vi "PicoScope6000aExampleStreamingQueue.vi"() -> ()   [LabVIEW 2015]
doc: "ps6000a Streaming example filling a single set of channel buffers at a time with LabVIEW queues."
uses:
  shared/PicoBuffers.ctl
  <vilib>/Waveform/DWDTOps.llb/DWDT Analog to Digital.vi
  PicoScope6000aLib/PicoScope6000aDigitalChannelSettings.ctl
  PicoScope6000aLib/PicoScope6000aAnalogChannelSettings.ctl
panel:
  in  "Poll Delay %":dbl=1.0 format="%#_13g"
  in  "Poll Holdoff %":dbl=90.0 format="%#_13g"
  out "Port 0":digitalwaveform(graph)={"t0"=timestamp(0 s since 1904-01-01), "dt"=1.004800013071339e-06, "Y"={"transitions"=[], "data"=[]}}
  out "Analog Channels":cluster{i32, dbl, "Data":dbl[]}[](graph)
  in  "Write ChA to file":bool
  out "Queue depth":i32(graph)
  out "queue depth":i32
  in  "Data file":path=path "PicoScope6000aExampleStreaming ChA Data"
  out "Max ADC value":i16
  out "DownSample Interval (sec)":dbl=1.0000000130088963e-06 format="%#.5p"
  out "Chunk time":u32
  out "Elapsed time":dbl
  in  "Auto Stop":bool
  in  "Apply Settings":bool
  in  "Channels":T1={"Channel A Settings "={"Enabled"=TRUE, "Coupling"=1, "Range"=0, "Analogue Offset"=0.0, "BandWidth"=0}, "Channel B Settings "={"Enabled"=FALSE, "Coupling"=1, "Range"=0, "Analogue Offset"=0.0, "BandWidth"=0}, "Channel C Settings "={"Enabled"=FALSE, "Coupling"=1, "Range"=0, "Analogue Offset"=0.0, "BandWidth"=0}, "Channel D Settings "={"Enabled"=FALSE, "Coupling"=1, "Range"=0, "Analogue Offset"=0.0, "BandWidth"=0}, "Channel E Settings "={"Enabled"=FALSE, "Coupling"=1, "Range"=0, "Analogue Offset"=0.0, "BandWidth"=0}, "Channel F Settings "={"Enabled"=FALSE, "Coupling"=1, "Range"=0, "Analogue Offset"=0.0, "BandWidth"=0}, "Channel G Settings "={"Enabled"=FALSE, "Coupling"=1, "Range"=0, "Analogue Offset"=0.0, "BandWidth"=0}, "Channel H Settings "={"Enabled"=FALSE, "Coupling"=1, "Range"=0, "Analogue Offset"=0.0, "BandWidth"=0}} {"Channel H Settings"."BandWidth" items=["Full"=0, "100kHz"=100000, "20kHz"=200000, "1MHz"=1000000, "20MHz"=20000000, "25MHz"=25000000, "50MHz"=50000000, "200MHz"=200000000, "250MHz"=250000000, "500MHz"=500000000]; "Channel H Settings"."Range" items=["10mV"=0, "20mV"=1, "50mV"=2, "100mV"=3, "200mV"=4, "500mV"=5, "1V"=6, "2V"=7, "5V"=8, "10V"=9, "20V"=10, "50V"=11, "100V"=12, "200V"=13, "x10_Probe_100mV"=32, "x10_Probe_200mV"=33, "x10_Probe_500mV"=34, "x10_Probe_1V"=35, "x10_Probe_2V"=36, "x10_Probe_5V"=37, "x10_Probe_10V"=38, "x10_Probe_20V"=39, "x10_Probe_50V"=40, "x10_Probe_100V"=41, "x10_Probe_200V"=42, "x10_Probe_500V"=43, "CURRENT_CLAMP_60A_2A"=10500, "CURRENT_CLAMP_60A_5A"=10501, "CURRENT_CLAMP_60A_10A"=10502, "CURRENT_CLAMP_60A_20A"=10503, "CURRENT_CLAMP_60A_50A"=10504, "CURRENT_CLAMP_60A_60A"=10505, "CURRENT_CLAMP_60A_V2_0_5A"=10600, "CURRENT_CLAMP_60A_V2_1A"=10601, "CURRENT_CLAMP_60A_V2_2A"=10602, "CURRENT_CLAMP_60A_V2_5A"=10603, "CURRENT_CLAMP_60A_V2_10A"=10604, "CURRENT_CLAMP_60A_V2_20A"=10605, "CURRENT_CLAMP_60A_V2_50A"=10606, "CURRENT_CLAMP_60A_V2_60A"=10607, "RESISTANCE_LEAD_NEG5_TO_20OHM"=7000, "RESISTANCE_LEAD_NEG50_TO_200OHM"=7001, "RESISTANCE_LEAD_NEG500_TO_2KOHM"=7002, "RESISTANCE_LEAD_NEG5K_TO_20KOHM"=7003, "RESISTANCE_LEAD_NEG50K_TO_LEAD_200KOHM"=7004, "RESISTANCE_LEAD_NEG500K_TO_LEAD_2MOHM"=7005, "RESISTANCE_LEAD_DIODE_TEST"=7006, "HT_NEG3_TO_5KV"=8950, "HT_NEG3_TO_10KV"=8951, "HT_NEG5_TO_20KV"=8952, "HT_NEG5_TO_50KV"=8953, "HT_NEG5_TO_100KV"=8954, "HT_NEG3_TO_5KV_INVERTED"=8955, "HT_NEG3_TO_10KV_INVERTED"=8956, "HT_NEG5_TO_20KV_INVERTED"=8957, "HT_NEG5_TO_50KV_INVERTED"=8958, "HT_NEG5_TO_100KV_INVERTED"=8959, "TEMPERATURE_NEG50_TO_150DEGC"=9000, "PRESSURE_SENSOR_-100k-150k_PASCALS"=9100, "PRESSURE_SENSOR_-100k_TO_400k_PASCALS"=9101, "PRESSURE_SENSOR_-200k_TO_800k_PASCALS"=9102, "PRESSURE_SENSOR_-400k_TO_1600k_PASCALS"=9103, "PRESSURE_SENSOR_-400k_TO_3400k_PASCALS"=9104, "PRESSURE_SENSOR_-150k_TO_1350k_PASCALS"=9105]; "Channel H Settings"."Coupling" items=["AC"=0, "DC 1M Ohm"=1, "DC 50 Ohm"=50]; "Channel G Settings"."BandWidth" items=["Full"=0, "100kHz"=100000, "20kHz"=200000, "1MHz"=1000000, "20MHz"=20000000, "25MHz"=25000000, "50MHz"=50000000, "200MHz"=200000000, "250MHz"=250000000, "500MHz"=500000000]; "Channel G Settings"."Range" items=["10mV"=0, "20mV"=1, "50mV"=2, "100mV"=3, "200mV"=4, "500mV"=5, "1V"=6, "2V"=7, "5V"=8, "10V"=9, "20V"=10, "50V"=11, "100V"=12, "200V"=13, "x10_Probe_100mV"=32, "x10_Probe_200mV"=33, "x10_Probe_500mV"=34, "x10_Probe_1V"=35, "x10_Probe_2V"=36, "x10_Probe_5V"=37, "x10_Probe_10V"=38, "x10_Probe_20V"=39, "x10_Probe_50V"=40, "x10_Probe_100V"=41, "x10_Probe_200V"=42, "x10_Probe_500V"=43, "CURRENT_CLAMP_60A_2A"=10500, "CURRENT_CLAMP_60A_5A"=10501, "CURRENT_CLAMP_60A_10A"=10502, "CURRENT_CLAMP_60A_20A"=10503, "CURRENT_CLAMP_60A_50A"=10504, "CURRENT_CLAMP_60A_60A"=10505, "CURRENT_CLAMP_60A_V2_0_5A"=10600, "CURRENT_CLAMP_60A_V2_1A"=10601, "CURRENT_CLAMP_60A_V2_2A"=10602, "CURRENT_CLAMP_60A_V2_5A"=10603, "CURRENT_CLAMP_60A_V2_10A"=10604, "CURRENT_CLAMP_60A_V2_20A"=10605, "CURRENT_CLAMP_60A_V2_50A"=10606, "CURRENT_CLAMP_60A_V2_60A"=10607, "RESISTANCE_LEAD_NEG5_TO_20OHM"=7000, "RESISTANCE_LEAD_NEG50_TO_200OHM"=7001, "RESISTANCE_LEAD_NEG500_TO_2KOHM"=7002, "RESISTANCE_LEAD_NEG5K_TO_20KOHM"=7003, "RESISTANCE_LEAD_NEG50K_TO_LEAD_200KOHM"=7004, "RESISTANCE_LEAD_NEG500K_TO_LEAD_2MOHM"=7005, "RESISTANCE_LEAD_DIODE_TEST"=7006, "HT_NEG3_TO_5KV"=8950, "HT_NEG3_TO_10KV"=8951, "HT_NEG5_TO_20KV"=8952, "HT_NEG5_TO_50KV"=8953, "HT_NEG5_TO_100KV"=8954, "HT_NEG3_TO_5KV_INVERTED"=8955, "HT_NEG3_TO_10KV_INVERTED"=8956, "HT_NEG5_TO_20KV_INVERTED"=8957, "HT_NEG5_TO_50KV_INVERTED"=8958, "HT_NEG5_TO_100KV_INVERTED"=8959, "TEMPERATURE_NEG50_TO_150DEGC"=9000, "PRESSURE_SENSOR_-100k-150k_PASCALS"=9100, "PRESSURE_SENSOR_-100k_TO_400k_PASCALS"=9101, "PRESSURE_SENSOR_-200k_TO_800k_PASCALS"=9102, "PRESSURE_SENSOR_-400k_TO_1600k_PASCALS"=9103, "PRESSURE_SENSOR_-400k_TO_3400k_PASCALS"=9104, "PRESSURE_SENSOR_-150k_TO_1350k_PASCALS"=9105]; "Channel G Settings"."Coupling" items=["AC"=0, "DC 1M Ohm"=1, "DC 50 Ohm"=50]; "Channel F Settings"."BandWidth" items=["Full"=0, "100kHz"=100000, "20kHz"=200000, "1MHz"=1000000, "20MHz"=20000000, "25MHz"=25000000, "50MHz"=50000000, "200MHz"=200000000, "250MHz"=250000000, "500MHz"=500000000]; "Channel F Settings"."Range" items=["10mV"=0, "20mV"=1, "50mV"=2, "100mV"=3, "200mV"=4, "500mV"=5, "1V"=6, "2V"=7, "5V"=8, "10V"=9, "20V"=10, "50V"=11, "100V"=12, "200V"=13, "x10_Probe_100mV"=32, "x10_Probe_200mV"=33, "x10_Probe_500mV"=34, "x10_Probe_1V"=35, "x10_Probe_2V"=36, "x10_Probe_5V"=37, "x10_Probe_10V"=38, "x10_Probe_20V"=39, "x10_Probe_50V"=40, "x10_Probe_100V"=41, "x10_Probe_200V"=42, "x10_Probe_500V"=43, "CURRENT_CLAMP_60A_2A"=10500, "CURRENT_CLAMP_60A_5A"=10501, "CURRENT_CLAMP_60A_10A"=10502, "CURRENT_CLAMP_60A_20A"=10503, "CURRENT_CLAMP_60A_50A"=10504, "CURRENT_CLAMP_60A_60A"=10505, "CURRENT_CLAMP_60A_V2_0_5A"=10600, "CURRENT_CLAMP_60A_V2_1A"=10601, "CURRENT_CLAMP_60A_V2_2A"=10602, "CURRENT_CLAMP_60A_V2_5A"=10603, "CURRENT_CLAMP_60A_V2_10A"=10604, "CURRENT_CLAMP_60A_V2_20A"=10605, "CURRENT_CLAMP_60A_V2_50A"=10606, "CURRENT_CLAMP_60A_V2_60A"=10607, "RESISTANCE_LEAD_NEG5_TO_20OHM"=7000, "RESISTANCE_LEAD_NEG50_TO_200OHM"=7001, "RESISTANCE_LEAD_NEG500_TO_2KOHM"=7002, "RESISTANCE_LEAD_NEG5K_TO_20KOHM"=7003, "RESISTANCE_LEAD_NEG50K_TO_LEAD_200KOHM"=7004, "RESISTANCE_LEAD_NEG500K_TO_LEAD_2MOHM"=7005, "RESISTANCE_LEAD_DIODE_TEST"=7006, "HT_NEG3_TO_5KV"=8950, "HT_NEG3_TO_10KV"=8951, "HT_NEG5_TO_20KV"=8952, "HT_NEG5_TO_50KV"=8953, "HT_NEG5_TO_100KV"=8954, "HT_NEG3_TO_5KV_INVERTED"=8955, "HT_NEG3_TO_10KV_INVERTED"=8956, "HT_NEG5_TO_20KV_INVERTED"=8957, "HT_NEG5_TO_50KV_INVERTED"=8958, "HT_NEG5_TO_100KV_INVERTED"=8959, "TEMPERATURE_NEG50_TO_150DEGC"=9000, "PRESSURE_SENSOR_-100k-150k_PASCALS"=9100, "PRESSURE_SENSOR_-100k_TO_400k_PASCALS"=9101, "PRESSURE_SENSOR_-200k_TO_800k_PASCALS"=9102, "PRESSURE_SENSOR_-400k_TO_1600k_PASCALS"=9103, "PRESSURE_SENSOR_-400k_TO_3400k_PASCALS"=9104, "PRESSURE_SENSOR_-150k_TO_1350k_PASCALS"=9105]; "Channel F Settings"."Coupling" items=["AC"=0, "DC 1M Ohm"=1, "DC 50 Ohm"=50]; "Channel E Settings"."BandWidth" items=["Full"=0, "100kHz"=100000, "20kHz"=200000, "1MHz"=1000000, "20MHz"=20000000, "25MHz"=25000000, "50MHz"=50000000, "200MHz"=200000000, "250MHz"=250000000, "500MHz"=500000000]; "Channel E Settings"."Range" items=["10mV"=0, "20mV"=1, "50mV"=2, "100mV"=3, "200mV"=4, "500mV"=5, "1V"=6, "2V"=7, "5V"=8, "10V"=9, "20V"=10, "50V"=11, "100V"=12, "200V"=13, "x10_Probe_100mV"=32, "x10_Probe_200mV"=33, "x10_Probe_500mV"=34, "x10_Probe_1V"=35, "x10_Probe_2V"=36, "x10_Probe_5V"=37, "x10_Probe_10V"=38, "x10_Probe_20V"=39, "x10_Probe_50V"=40, "x10_Probe_100V"=41, "x10_Probe_200V"=42, "x10_Probe_500V"=43, "CURRENT_CLAMP_60A_2A"=10500, "CURRENT_CLAMP_60A_5A"=10501, "CURRENT_CLAMP_60A_10A"=10502, "CURRENT_CLAMP_60A_20A"=10503, "CURRENT_CLAMP_60A_50A"=10504, "CURRENT_CLAMP_60A_60A"=10505, "CURRENT_CLAMP_60A_V2_0_5A"=10600, "CURRENT_CLAMP_60A_V2_1A"=10601, "CURRENT_CLAMP_60A_V2_2A"=10602, "CURRENT_CLAMP_60A_V2_5A"=10603, "CURRENT_CLAMP_60A_V2_10A"=10604, "CURRENT_CLAMP_60A_V2_20A"=10605, "CURRENT_CLAMP_60A_V2_50A"=10606, "CURRENT_CLAMP_60A_V2_60A"=10607, "RESISTANCE_LEAD_NEG5_TO_20OHM"=7000, "RESISTANCE_LEAD_NEG50_TO_200OHM"=7001, "RESISTANCE_LEAD_NEG500_TO_2KOHM"=7002, "RESISTANCE_LEAD_NEG5K_TO_20KOHM"=7003, "RESISTANCE_LEAD_NEG50K_TO_LEAD_200KOHM"=7004, "RESISTANCE_LEAD_NEG500K_TO_LEAD_2MOHM"=7005, "RESISTANCE_LEAD_DIODE_TEST"=7006, "HT_NEG3_TO_5KV"=8950, "HT_NEG3_TO_10KV"=8951, "HT_NEG5_TO_20KV"=8952, "HT_NEG5_TO_50KV"=8953, "HT_NEG5_TO_100KV"=8954, "HT_NEG3_TO_5KV_INVERTED"=8955, "HT_NEG3_TO_10KV_INVERTED"=8956, "HT_NEG5_TO_20KV_INVERTED"=8957, "HT_NEG5_TO_50KV_INVERTED"=8958, "HT_NEG5_TO_100KV_INVERTED"=8959, "TEMPERATURE_NEG50_TO_150DEGC"=9000, "PRESSURE_SENSOR_-100k-150k_PASCALS"=9100, "PRESSURE_SENSOR_-100k_TO_400k_PASCALS"=9101, "PRESSURE_SENSOR_-200k_TO_800k_PASCALS"=9102, "PRESSURE_SENSOR_-400k_TO_1600k_PASCALS"=9103, "PRESSURE_SENSOR_-400k_TO_3400k_PASCALS"=9104, "PRESSURE_SENSOR_-150k_TO_1350k_PASCALS"=9105]; "Channel E Settings"."Coupling" items=["AC"=0, "DC 1M Ohm"=1, "DC 50 Ohm"=50]; "Channel D Settings"."BandWidth" items=["Full"=0, "100kHz"=100000, "20kHz"=200000, "1MHz"=1000000, "20MHz"=20000000, "25MHz"=25000000, "50MHz"=50000000, "200MHz"=200000000, "250MHz"=250000000, "500MHz"=500000000]; "Channel D Settings"."Range" items=["10mV"=0, "20mV"=1, "50mV"=2, "100mV"=3, "200mV"=4, "500mV"=5, "1V"=6, "2V"=7, "5V"=8, "10V"=9, "20V"=10, "50V"=11, "100V"=12, "200V"=13, "x10_Probe_100mV"=32, "x10_Probe_200mV"=33, "x10_Probe_500mV"=34, "x10_Probe_1V"=35, "x10_Probe_2V"=36, "x10_Probe_5V"=37, "x10_Probe_10V"=38, "x10_Probe_20V"=39, "x10_Probe_50V"=40, "x10_Probe_100V"=41, "x10_Probe_200V"=42, "x10_Probe_500V"=43, "CURRENT_CLAMP_60A_2A"=10500, "CURRENT_CLAMP_60A_5A"=10501, "CURRENT_CLAMP_60A_10A"=10502, "CURRENT_CLAMP_60A_20A"=10503, "CURRENT_CLAMP_60A_50A"=10504, "CURRENT_CLAMP_60A_60A"=10505, "CURRENT_CLAMP_60A_V2_0_5A"=10600, "CURRENT_CLAMP_60A_V2_1A"=10601, "CURRENT_CLAMP_60A_V2_2A"=10602, "CURRENT_CLAMP_60A_V2_5A"=10603, "CURRENT_CLAMP_60A_V2_10A"=10604, "CURRENT_CLAMP_60A_V2_20A"=10605, "CURRENT_CLAMP_60A_V2_50A"=10606, "CURRENT_CLAMP_60A_V2_60A"=10607, "RESISTANCE_LEAD_NEG5_TO_20OHM"=7000, "RESISTANCE_LEAD_NEG50_TO_200OHM"=7001, "RESISTANCE_LEAD_NEG500_TO_2KOHM"=7002, "RESISTANCE_LEAD_NEG5K_TO_20KOHM"=7003, "RESISTANCE_LEAD_NEG50K_TO_LEAD_200KOHM"=7004, "RESISTANCE_LEAD_NEG500K_TO_LEAD_2MOHM"=7005, "RESISTANCE_LEAD_DIODE_TEST"=7006, "HT_NEG3_TO_5KV"=8950, "HT_NEG3_TO_10KV"=8951, "HT_NEG5_TO_20KV"=8952, "HT_NEG5_TO_50KV"=8953, "HT_NEG5_TO_100KV"=8954, "HT_NEG3_TO_5KV_INVERTED"=8955, "HT_NEG3_TO_10KV_INVERTED"=8956, "HT_NEG5_TO_20KV_INVERTED"=8957, "HT_NEG5_TO_50KV_INVERTED"=8958, "HT_NEG5_TO_100KV_INVERTED"=8959, "TEMPERATURE_NEG50_TO_150DEGC"=9000, "PRESSURE_SENSOR_-100k-150k_PASCALS"=9100, "PRESSURE_SENSOR_-100k_TO_400k_PASCALS"=9101, "PRESSURE_SENSOR_-200k_TO_800k_PASCALS"=9102, "PRESSURE_SENSOR_-400k_TO_1600k_PASCALS"=9103, "PRESSURE_SENSOR_-400k_TO_3400k_PASCALS"=9104, "PRESSURE_SENSOR_-150k_TO_1350k_PASCALS"=9105]; "Channel D Settings"."Coupling" items=["AC"=0, "DC 1M Ohm"=1, "DC 50 Ohm"=50]; "Channel C Settings"."BandWidth" items=["Full"=0, "100kHz"=100000, "20kHz"=200000, "1MHz"=1000000, "20MHz"=20000000, "25MHz"=25000000, "50MHz"=50000000, "200MHz"=200000000, "250MHz"=250000000, "500MHz"=500000000]; "Channel C Settings"."Range" items=["10mV"=0, "20mV"=1, "50mV"=2, "100mV"=3, "200mV"=4, "500mV"=5, "1V"=6, "2V"=7, "5V"=8, "10V"=9, "20V"=10, "50V"=11, "100V"=12, "200V"=13, "x10_Probe_100mV"=32, "x10_Probe_200mV"=33, "x10_Probe_500mV"=34, "x10_Probe_1V"=35, "x10_Probe_2V"=36, "x10_Probe_5V"=37, "x10_Probe_10V"=38, "x10_Probe_20V"=39, "x10_Probe_50V"=40, "x10_Probe_100V"=41, "x10_Probe_200V"=42, "x10_Probe_500V"=43, "CURRENT_CLAMP_60A_2A"=10500, "CURRENT_CLAMP_60A_5A"=10501, "CURRENT_CLAMP_60A_10A"=10502, "CURRENT_CLAMP_60A_20A"=10503, "CURRENT_CLAMP_60A_50A"=10504, "CURRENT_CLAMP_60A_60A"=10505, "CURRENT_CLAMP_60A_V2_0_5A"=10600, "CURRENT_CLAMP_60A_V2_1A"=10601, "CURRENT_CLAMP_60A_V2_2A"=10602, "CURRENT_CLAMP_60A_V2_5A"=10603, "CURRENT_CLAMP_60A_V2_10A"=10604, "CURRENT_CLAMP_60A_V2_20A"=10605, "CURRENT_CLAMP_60A_V2_50A"=10606, "CURRENT_CLAMP_60A_V2_60A"=10607, "RESISTANCE_LEAD_NEG5_TO_20OHM"=7000, "RESISTANCE_LEAD_NEG50_TO_200OHM"=7001, "RESISTANCE_LEAD_NEG500_TO_2KOHM"=7002, "RESISTANCE_LEAD_NEG5K_TO_20KOHM"=7003, "RESISTANCE_LEAD_NEG50K_TO_LEAD_200KOHM"=7004, "RESISTANCE_LEAD_NEG500K_TO_LEAD_2MOHM"=7005, "RESISTANCE_LEAD_DIODE_TEST"=7006, "HT_NEG3_TO_5KV"=8950, "HT_NEG3_TO_10KV"=8951, "HT_NEG5_TO_20KV"=8952, "HT_NEG5_TO_50KV"=8953, "HT_NEG5_TO_100KV"=8954, "HT_NEG3_TO_5KV_INVERTED"=8955, "HT_NEG3_TO_10KV_INVERTED"=8956, "HT_NEG5_TO_20KV_INVERTED"=8957, "HT_NEG5_TO_50KV_INVERTED"=8958, "HT_NEG5_TO_100KV_INVERTED"=8959, "TEMPERATURE_NEG50_TO_150DEGC"=9000, "PRESSURE_SENSOR_-100k-150k_PASCALS"=9100, "PRESSURE_SENSOR_-100k_TO_400k_PASCALS"=9101, "PRESSURE_SENSOR_-200k_TO_800k_PASCALS"=9102, "PRESSURE_SENSOR_-400k_TO_1600k_PASCALS"=9103, "PRESSURE_SENSOR_-400k_TO_3400k_PASCALS"=9104, "PRESSURE_SENSOR_-150k_TO_1350k_PASCALS"=9105]; "Channel C Settings"."Coupling" items=["AC"=0, "DC 1M Ohm"=1, "DC 50 Ohm"=50]; "Channel B Settings"."BandWidth" items=["Full"=0, "100kHz"=100000, "20kHz"=200000, "1MHz"=1000000, "20MHz"=20000000, "25MHz"=25000000, "50MHz"=50000000, "200MHz"=200000000, "250MHz"=250000000, "500MHz"=500000000]; "Channel B Settings"."Range" items=["10mV"=0, "20mV"=1, "50mV"=2, "100mV"=3, "200mV"=4, "500mV"=5, "1V"=6, "2V"=7, "5V"=8, "10V"=9, "20V"=10, "50V"=11, "100V"=12, "200V"=13, "x10_Probe_100mV"=32, "x10_Probe_200mV"=33, "x10_Probe_500mV"=34, "x10_Probe_1V"=35, "x10_Probe_2V"=36, "x10_Probe_5V"=37, "x10_Probe_10V"=38, "x10_Probe_20V"=39, "x10_Probe_50V"=40, "x10_Probe_100V"=41, "x10_Probe_200V"=42, "x10_Probe_500V"=43, "CURRENT_CLAMP_60A_2A"=10500, "CURRENT_CLAMP_60A_5A"=10501, "CURRENT_CLAMP_60A_10A"=10502, "CURRENT_CLAMP_60A_20A"=10503, "CURRENT_CLAMP_60A_50A"=10504, "CURRENT_CLAMP_60A_60A"=10505, "CURRENT_CLAMP_60A_V2_0_5A"=10600, "CURRENT_CLAMP_60A_V2_1A"=10601, "CURRENT_CLAMP_60A_V2_2A"=10602, "CURRENT_CLAMP_60A_V2_5A"=10603, "CURRENT_CLAMP_60A_V2_10A"=10604, "CURRENT_CLAMP_60A_V2_20A"=10605, "CURRENT_CLAMP_60A_V2_50A"=10606, "CURRENT_CLAMP_60A_V2_60A"=10607, "RESISTANCE_LEAD_NEG5_TO_20OHM"=7000, "RESISTANCE_LEAD_NEG50_TO_200OHM"=7001, "RESISTANCE_LEAD_NEG500_TO_2KOHM"=7002, "RESISTANCE_LEAD_NEG5K_TO_20KOHM"=7003, "RESISTANCE_LEAD_NEG50K_TO_LEAD_200KOHM"=7004, "RESISTANCE_LEAD_NEG500K_TO_LEAD_2MOHM"=7005, "RESISTANCE_LEAD_DIODE_TEST"=7006, "HT_NEG3_TO_5KV"=8950, "HT_NEG3_TO_10KV"=8951, "HT_NEG5_TO_20KV"=8952, "HT_NEG5_TO_50KV"=8953, "HT_NEG5_TO_100KV"=8954, "HT_NEG3_TO_5KV_INVERTED"=8955, "HT_NEG3_TO_10KV_INVERTED"=8956, "HT_NEG5_TO_20KV_INVERTED"=8957, "HT_NEG5_TO_50KV_INVERTED"=8958, "HT_NEG5_TO_100KV_INVERTED"=8959, "TEMPERATURE_NEG50_TO_150DEGC"=9000, "PRESSURE_SENSOR_-100k-150k_PASCALS"=9100, "PRESSURE_SENSOR_-100k_TO_400k_PASCALS"=9101, "PRESSURE_SENSOR_-200k_TO_800k_PASCALS"=9102, "PRESSURE_SENSOR_-400k_TO_1600k_PASCALS"=9103, "PRESSURE_SENSOR_-400k_TO_3400k_PASCALS"=9104, "PRESSURE_SENSOR_-150k_TO_1350k_PASCALS"=9105]; "Channel B Settings"."Coupling" items=["AC"=0, "DC 1M Ohm"=1, "DC 50 Ohm"=50]; "Channel A Settings"."Range" items=["10mV"=0, "20mV"=1, "50mV"=2, "100mV"=3, "200mV"=4, "500mV"=5, "1V"=6, "2V"=7, "5V"=8, "10V"=9, "20V"=10, "50V"=11, "100V"=12, "200V"=13, "x10_Probe_100mV"=32, "x10_Probe_200mV"=33, "x10_Probe_500mV"=34, "x10_Probe_1V"=35, "x10_Probe_2V"=36, "x10_Probe_5V"=37, "x10_Probe_10V"=38, "x10_Probe_20V"=39, "x10_Probe_50V"=40, "x10_Probe_100V"=41, "x10_Probe_200V"=42, "x10_Probe_500V"=43, "CURRENT_CLAMP_60A_2A"=10500, "CURRENT_CLAMP_60A_5A"=10501, "CURRENT_CLAMP_60A_10A"=10502, "CURRENT_CLAMP_60A_20A"=10503, "CURRENT_CLAMP_60A_50A"=10504, "CURRENT_CLAMP_60A_60A"=10505, "CURRENT_CLAMP_60A_V2_0_5A"=10600, "CURRENT_CLAMP_60A_V2_1A"=10601, "CURRENT_CLAMP_60A_V2_2A"=10602, "CURRENT_CLAMP_60A_V2_5A"=10603, "CURRENT_CLAMP_60A_V2_10A"=10604, "CURRENT_CLAMP_60A_V2_20A"=10605, "CURRENT_CLAMP_60A_V2_50A"=10606, "CURRENT_CLAMP_60A_V2_60A"=10607, "RESISTANCE_LEAD_NEG5_TO_20OHM"=7000, "RESISTANCE_LEAD_NEG50_TO_200OHM"=7001, "RESISTANCE_LEAD_NEG500_TO_2KOHM"=7002, "RESISTANCE_LEAD_NEG5K_TO_20KOHM"=7003, "RESISTANCE_LEAD_NEG50K_TO_LEAD_200KOHM"=7004, "RESISTANCE_LEAD_NEG500K_TO_LEAD_2MOHM"=7005, "RESISTANCE_LEAD_DIODE_TEST"=7006, "HT_NEG3_TO_5KV"=8950, "HT_NEG3_TO_10KV"=8951, "HT_NEG5_TO_20KV"=8952, "HT_NEG5_TO_50KV"=8953, "HT_NEG5_TO_100KV"=8954, "HT_NEG3_TO_5KV_INVERTED"=8955, "HT_NEG3_TO_10KV_INVERTED"=8956, "HT_NEG5_TO_20KV_INVERTED"=8957, "HT_NEG5_TO_50KV_INVERTED"=8958, "HT_NEG5_TO_100KV_INVERTED"=8959, "TEMPERATURE_NEG50_TO_150DEGC"=9000, "PRESSURE_SENSOR_-100k-150k_PASCALS"=9100, "PRESSURE_SENSOR_-100k_TO_400k_PASCALS"=9101, "PRESSURE_SENSOR_-200k_TO_800k_PASCALS"=9102, "PRESSURE_SENSOR_-400k_TO_1600k_PASCALS"=9103, "PRESSURE_SENSOR_-400k_TO_3400k_PASCALS"=9104, "PRESSURE_SENSOR_-150k_TO_1350k_PASCALS"=9105]; "Channel A Settings"."BandWidth" items=["Full"=0, "100kHz"=100000, "20kHz"=200000, "1MHz"=1000000, "20MHz"=20000000, "25MHz"=25000000, "50MHz"=50000000, "200MHz"=200000000, "250MHz"=250000000, "500MHz"=500000000]; "Channel A Settings"."Coupling" items=["AC"=0, "DC 1M Ohm"=1, "DC 50 Ohm"=50]}
  in  "Digital Channels":T2={"Port 0 Settings "={"Enabled"=FALSE, "Hysteresis"=3, "Threshold Level (Volts)"=[1.0, 1.0, 1.0, 1.0, 1.0, 1.0, 1.0, 1.0]}, "Port 1 Settings"={"Enabled"=FALSE, "Hysteresis"=3, "Threshold Level (Volts)"=[1.0, 1.0, 1.0, 1.0, 1.0, 1.0, 1.0, 1.0]}} {"Port 1 Settings"."Threshold Level (Volts)" format="%#_4p"; "Port 1 Settings"."Hysteresis" items=["PICO_VERY_HIGH_400MV", "PICO_HIGH_200MV", "PICO_NORMAL_100MV", "PICO_LOW_50MV"]; "Port 0 Settings"."Threshold Level (Volts)" format="%#_4p"; "Port 0 Settings"."Hysteresis" items=["PICO_VERY_HIGH_400MV", "PICO_HIGH_200MV", "PICO_NORMAL_100MV", "PICO_LOW_50MV"]}
  in  "No of Buffers":i32=2 min=2
  in  "Streaming Acquisition Settings":T3={"preTriggerSamples"=0, "postTriggerSamples"=100000, "Requested sampleInterval"=1.0, "sampleIntervalTimeUnits"=3} {"sampleIntervalTimeUnits" items=["femtoseconds", "picoseconds", "nanoseconds", "microseconds", "millseconds", "seconds"]; "postTriggerSamples" format="%_6p"; "preTriggerSamples" format="%_6p"}
  in  "Buffer and Transfer Settings":T4={"startIndex"=0, "Samples"=100000, "Down Sample Ratio"=1, "Down-Sample Mode"=2147483648} {"Down-Sample Mode" items=["None"=2147483648, "Aggregate"=1, "Decimate"=2, "Average"=4]; "Down Sample Ratio" step=1; "Samples" format="%_6p"}
  in  "Trigger Settings":T5={"Trigger Enabled"=FALSE, "Trigger Threshold (Volts)"=0.0, "Trigger Direction"=2, "Trigger Delay (samples)"=0, "Auto Trigger Time (us)"=100000, "Trigger Source"=0} {"Trigger Source" items=["Channel A"=0, "Channel B"=1, "Channel C"=2, "Channel D"=3, "Channel E"=4, "Channel F"=5, "Channel G"=6, "Channel H"=7, "Port 0"=128, "Port 1"=129, "Trigger AUX"=1001]; "Trigger Direction" items=["Rising"=2, "Falling"=3]; "Trigger Threshold (Volts)" format="%#_6p"}
  in  "stop":bool
  out "Device Info":T6={"PICO_DRIVER_VERSION"="ps6000a Windows Driver, 1.0.82.3072", "PICO_USB_VERSION"="3.0", "PICO_HARDWARE_VERSION"="1.1", "PICO_VARIANT_INFO"="6824E", "PICO_BATCH_AND_SERIAL"="FU811/0026", "PICO_CAL_DATE"="06Dec19", "PICO_KERNEL_VERSION"="1.0", "PICO_DIGITAL_HARDWARE_VERSION"="1", "PICO_ANALOGUE_HARDWARE_VERSION"="1", "PICO_FIRMWARE_VERSION_1"="1.7.16.0", "PICO_FIRMWARE_VERSION_2"="1.1.4.0", "PICO_IPP_VERSION"="1.4.0-133", "PICO_DRIVER_PATH"="C:\\Program Files\\Pico Technology\\SDK\\lib\\ps6000a.dll", "PICO_FIRMWARE_VERSION_3"="1.1.49.0", "PICO_FRONT_PANEL_FIRMWARE_VERSION"="1.0.0.0", "Number of Channels"=8, "MSO"=TRUE}
  out "Pico 6000a Units":string
  in  "Resolution":u32(ring) items=["8-bit"=0, "12-bit"=1, "14-bit"=2, "15-bit"=3, "16-bit"=4, "10-bit"=10]
  in  "Serial Number":string
  in  "Use Serial Number":bool
  in  "error in (no error)":errorcluster
  # "D8-D15"
  # "DO-D7"
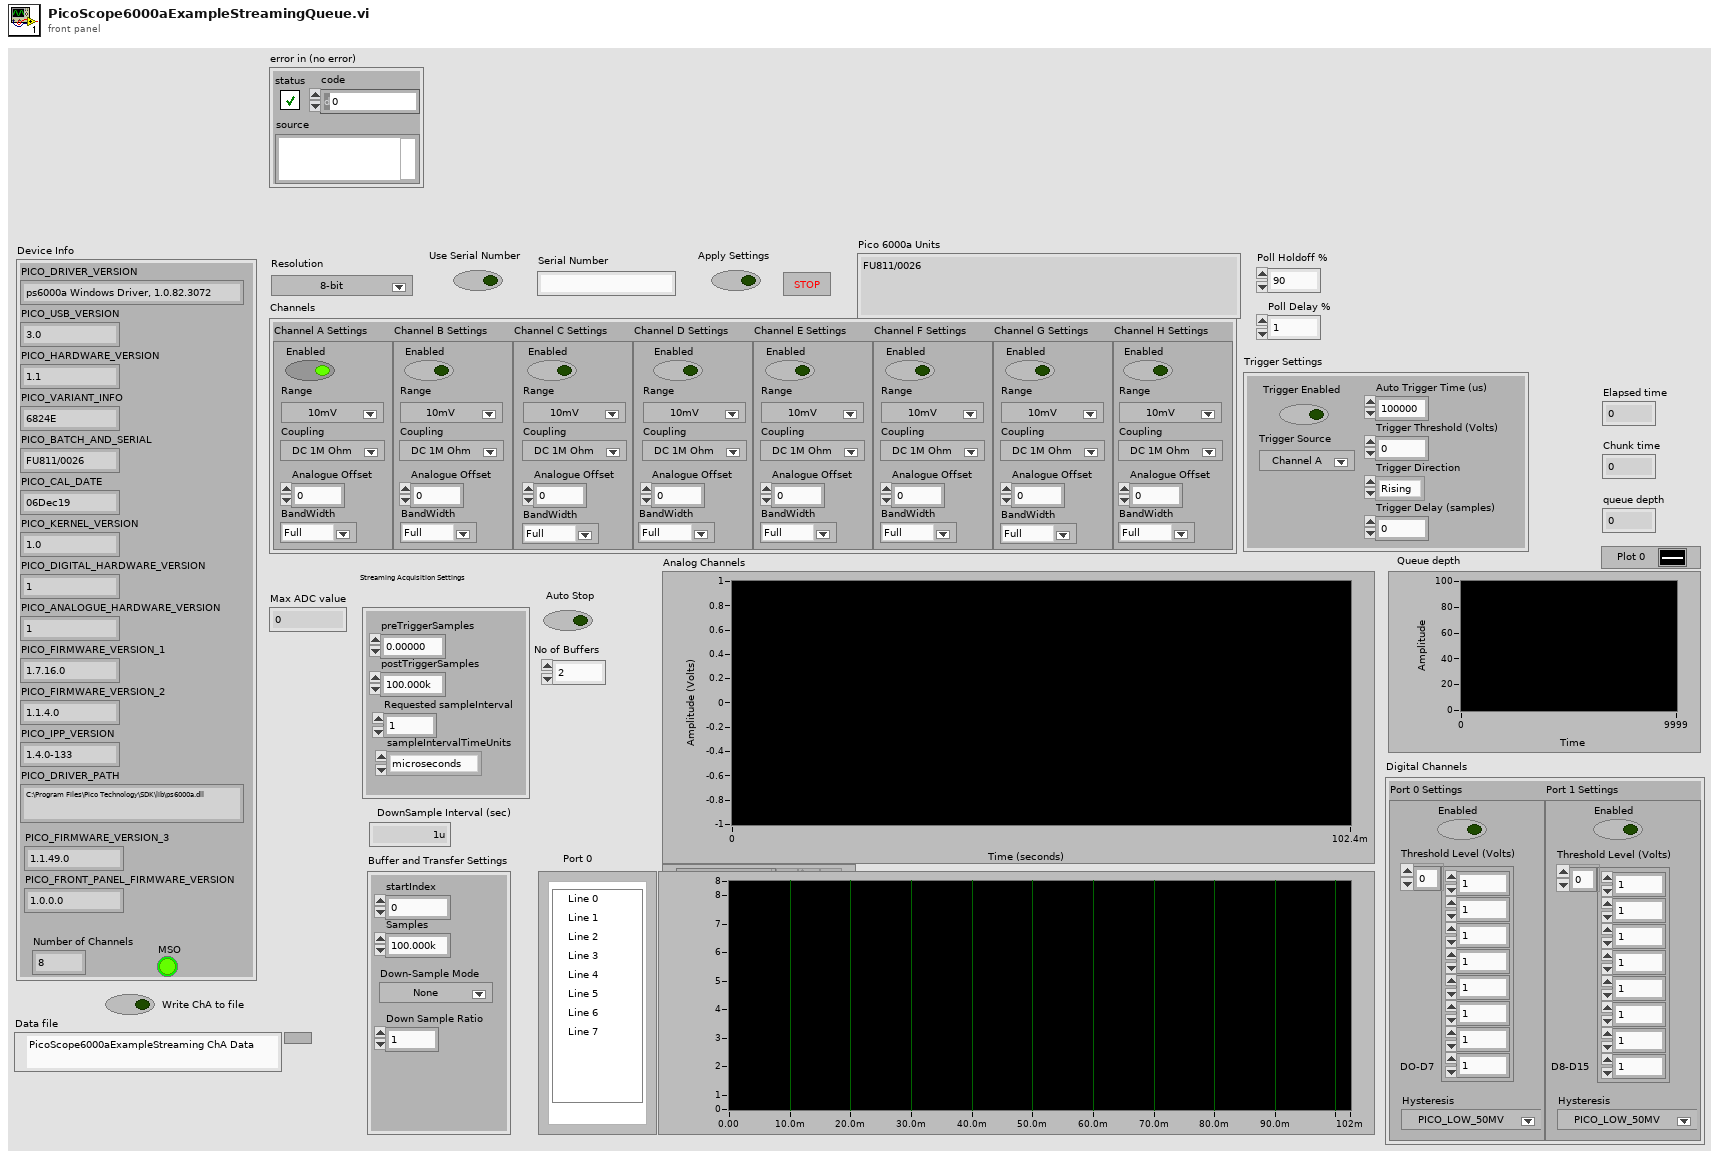
[diagram p1: front panel]
types:
  T1 = typedef "PicoScope6000aAnalogChannelSettings.ctl" = cluster{"Channel A Settings ":cluster{"Enabled":bool, "Coupling":i16, "Range":u16, "Analogue Offset":dbl, "BandWidth":u32}, "Channel B Settings ":cluster{"Enabled":bool, "Coupling":i16, "Range":u16, "Analogue Offset":dbl, "BandWidth":u32}, "Channel C Settings ":cluster{"Enabled":bool, "Coupling":i16, "Range":u16, "Analogue Offset":dbl, "BandWidth":u32}, "Channel D Settings ":cluster{"Enabled":bool, "Coupling":i16, "Range":u16, "Analogue Offset":dbl, "BandWidth":u32}, "Channel E Settings ":cluster{"Enabled":bool, "Coupling":i16, "Range":u16, "Analogue Offset":dbl, "BandWidth":u32}, "Channel F Settings ":cluster{"Enabled":bool, "Coupling":i16, "Range":u16, "Analogue Offset":dbl, "BandWidth":u32}, "Channel G Settings ":cluster{"Enabled":bool, "Coupling":i16, "Range":u16, "Analogue Offset":dbl, "BandWidth":u32}, "Channel H Settings ":cluster{"Enabled":bool, "Coupling":i16, "Range":u16, "Analogue Offset":dbl, "BandWidth":u32}}
  T2 = typedef "PicoScope6000aDigitalChannelSettings.ctl" = cluster{"Port 0 Settings ":cluster{"Enabled":bool, "Hysteresis":u32, "Threshold Level (Volts)":dbl[]}, "Port 1 Settings":cluster{"Enabled":bool, "Hysteresis":u32, "Threshold Level (Volts)":dbl[]}}
  T3 = cluster{"preTriggerSamples":u64, "postTriggerSamples":u64, "Requested sampleInterval":dbl, "sampleIntervalTimeUnits":u32}
  T4 = cluster{"startIndex":u64, "Samples":u64, "Down Sample Ratio":u64, "Down-Sample Mode":u32}
  T5 = cluster{"Trigger Enabled":bool, "Trigger Threshold (Volts)":dbl, "Trigger Direction":u16, "Trigger Delay (samples)":u64, "Auto Trigger Time (us)":u32, "Trigger Source":u32}
  T6 = cluster{"PICO_DRIVER_VERSION":string, "PICO_USB_VERSION":string, "PICO_HARDWARE_VERSION":string, "PICO_VARIANT_INFO":string, "PICO_BATCH_AND_SERIAL":string, "PICO_CAL_DATE":string, "PICO_KERNEL_VERSION":string, "PICO_DIGITAL_HARDWARE_VERSION":string, "PICO_ANALOGUE_HARDWARE_VERSION":string, "PICO_FIRMWARE_VERSION_1":string, "PICO_FIRMWARE_VERSION_2":string, "PICO_IPP_VERSION":string, "PICO_DRIVER_PATH":string, "PICO_FIRMWARE_VERSION_3":string, "PICO_FRONT_PANEL_FIRMWARE_VERSION":string, "Number of Channels":i16, "MSO":bool}
  T7 = typedef "PicoBuffers.ctl" = cluster{"Max Buffer Pointers":u64[][][], "Min Buffer Pointers":u64[][][], "StreamingDataInfo":cluster{"Channel":u32, "Down-Sample Mode":u32, "PICO_DATA_TYPE":enum32{"PICO_INT8_T", "PICO_INT16_T", "PICO_INT32_T", "PICO_UINT32_T", "PICO_INT64_T", ""}, "Samples":i32, "bufferIndex":u64, "startIndex":i32, "overflow":i16}[][]}
  T8 = enum16{"open", "open or create", "create or replace", "create", "open (read-only)"}
  T9 = cluster{i32, "DownSample Interval (sec)":dbl, "Data":dbl[]}
  T10 = cluster{i32, "DownSample Interval (sec)":dbl, "Data":dbl[]}[]
  T11 = cluster{"sampleInterval":dbl, "sampleIntervalTimeUnits":u32}
  T12 = cluster{"triggerAt_":u64, "triggered_":i16, "autoStop_":i16}
  T13 = cluster{"Channel A Buffer":i16[], "Channel B Buffer":i16[], "Channel C Buffer":i16[], "Channel D Buffer":i16[], "Channel E Buffer":i16[], "Channel F Buffer":i16[], "Channel G Buffer":i16[], "Channel H Buffer":i16[], "Port 0 Buffer":i16[], "Port 1 Buffer":i16[]}
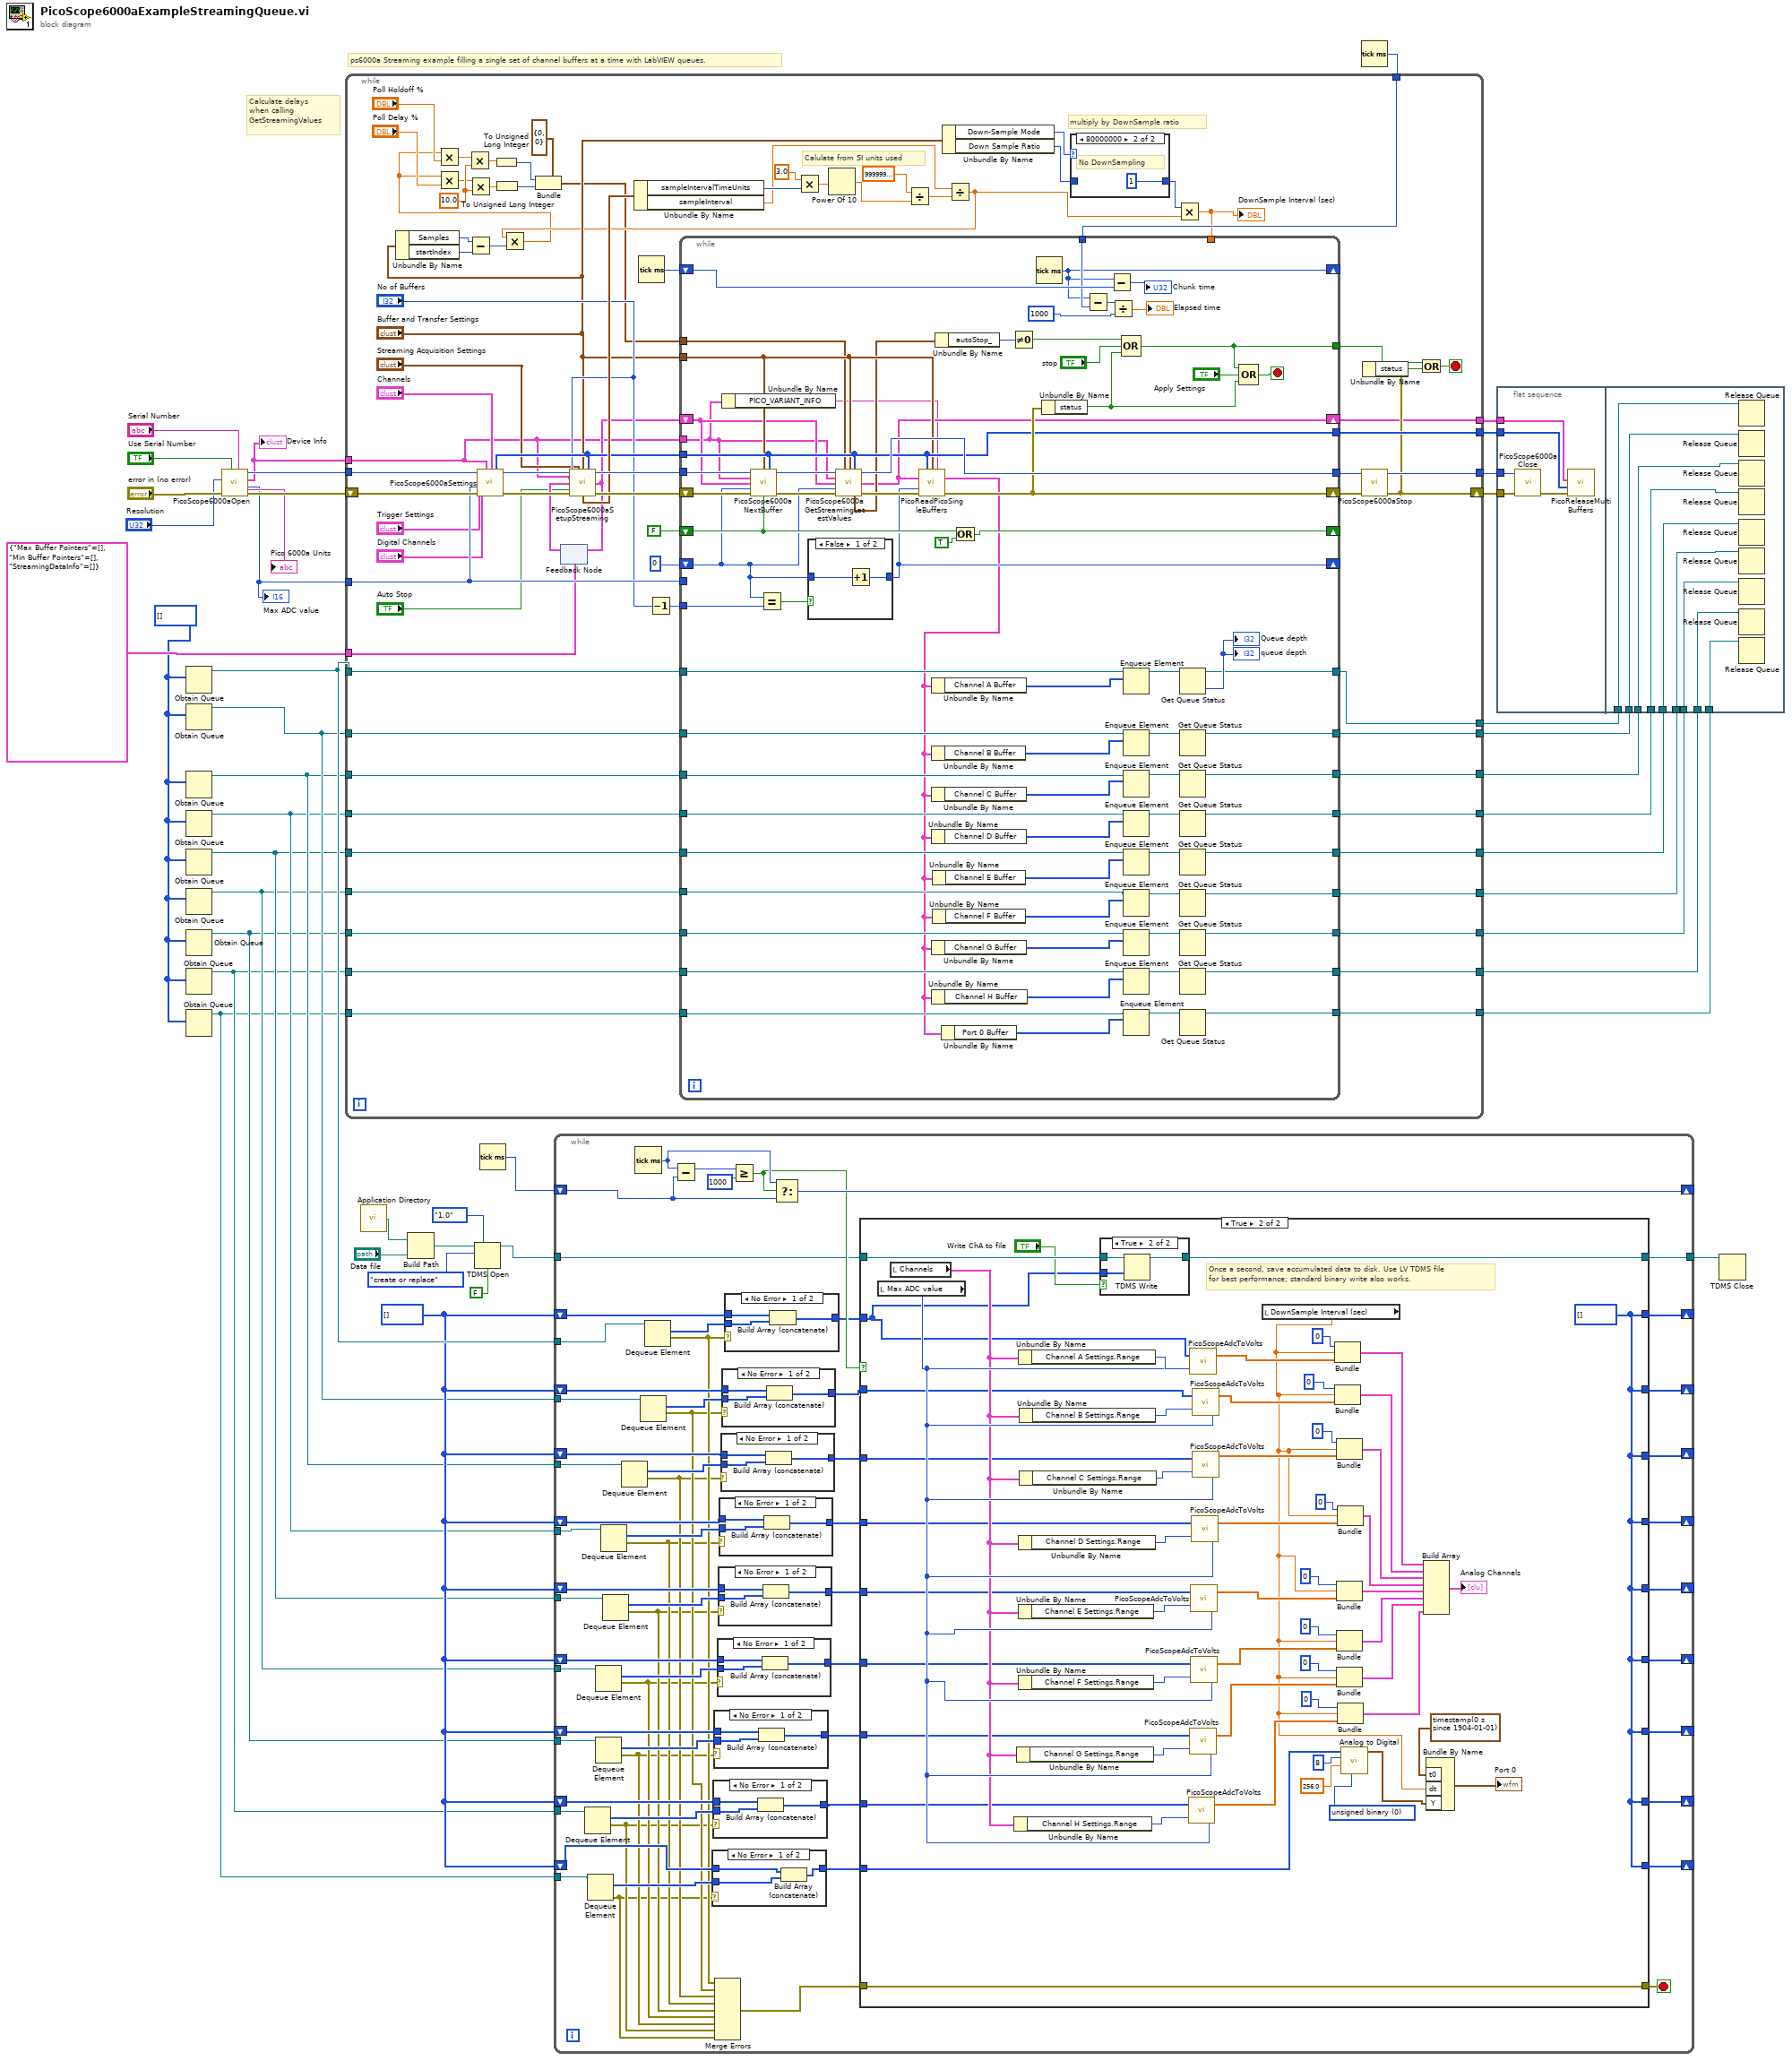
[diagram p0: block diagram]
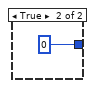
[diagram p13: hidden frame]
diagram:
  w16 = i16[] [] ("History Data")
  w17 = i16[] [] ("History Data")
  # "Calculate delays\nwhen calling\nGetStreamingValues"
  # "ps6000a Streaming example filling a single set of channel buffers at a time with LabVIEW queues."
  n1 = Obtain Queue(element data type=w16) -> (queue out=w19:refnum<queue>)  [unwired: 4 in, 2 out]
  n2 = Obtain Queue(element data type=w16) -> (queue out=w15:refnum<queue>)  [unwired: 4 in, 2 out]
  n3 = Obtain Queue(element data type=w16) -> (queue out=w14:refnum<queue>)  [unwired: 4 in, 2 out]
  n4 = Obtain Queue(element data type=w16) -> (queue out=w13:refnum<queue>)  [unwired: 4 in, 2 out]
  n5 = Obtain Queue(element data type=w16) -> (queue out=w12:refnum<queue>)  [unwired: 4 in, 2 out]
  n6 = Obtain Queue(element data type=w16) -> (queue out=w11:refnum<queue>)  [unwired: 4 in, 2 out]
  n7 = Obtain Queue(element data type=w16) -> (queue out=w10:refnum<queue>)  [unwired: 4 in, 2 out]
  n8 = Obtain Queue(element data type=w16) -> (queue out=w9:refnum<queue>)  [unwired: 4 in, 2 out]
  n9 = Obtain Queue(element data type=w16) -> (queue out=w8:refnum<queue>)  [unwired: 4 in, 2 out]
  n10 = call "PicoScope6000aOpen.vi"("Serial Number"="Serial Number", "Use Serial Number"="Use Serial Number", "error in (no error)"="error in (no error)", "Resolution"="Resolution") -> ("error out"=w40:errorcluster, "Max ADC value"=w26:i16, "Device Info"=w37:T6, "handle out"=w41:i16, "Pico 6000a Units"=→"Pico 6000a Units":string)  [unwired: 2 in, 1 out]
  "Device Info" <- w37
  "Max ADC value" <- w26
  n11 = call <vilib>:"Application Directory.vi"() -> ("Application Directory"=w27:path)
  n12 = Build Path(base path=w27, name or relative path="Data file") -> (appended path=w28:path)
  n13 = TDMS Open(6:FALSE ("disable buffering? (T)"), 7:enum16{"1.0", "2.0"}."1.0" ("file format version (2.0)"), 10:T8."create or replace" ("operation (0:open)"), 11:w28) -> (3:w33:refnum<k34>)  [unwired: 3 in, 1 out]
  n14 = Tick Count (ms)() -> (millisecond timer value=w35:u32)
  n15 = while {
    tunnel: w19 -> [w107]
    shift-right: [w98] -> _
    shift-left: w17 -> [w106]
    shift-right: [w101] -> _
    shift-left: w35 -> [w102]
    tunnel: w33 -> [w97]
    tunnel: [w96] -> w32
    shift-right: [w92] -> _
    shift-left: w17 -> [w94]
    shift-right: [w81] -> _
    shift-left: w17 -> [w82]
    shift-right: [w78] -> _
    shift-left: w17 -> [w79]
    shift-right: [w71] -> _
    shift-left: w17 -> [w76]
    shift-right: [w70] -> _
    shift-left: w17 -> [w75]
    shift-right: [w69] -> _
    shift-left: w17 -> [w74]
    shift-right: [w68] -> _
    shift-left: w17 -> [w73]
    shift-right: [w67] -> _
    shift-left: w17 -> [w72]
    tunnel: w15 -> [w52]
    tunnel: w14 -> [w51]
    tunnel: w13 -> [w50]
    tunnel: w12 -> [w49]
    tunnel: w11 -> [w48]
    tunnel: w10 -> [w47]
    tunnel: w9 -> [w46]
    tunnel: w8 -> [w45]
    stop <- w91 stop-if-true
    n16 = Dequeue Element(queue=w46) -> (element=w83:i16[], error out=w54:errorcluster)  [unwired: 2 in, 2 out]
    n17 = Dequeue Element(queue=w45) -> (element=w95:i16[], error out=w53:errorcluster)  [unwired: 2 in, 2 out]
    n18 = Dequeue Element(queue=w48) -> (element=w85:i16[], error out=w56:errorcluster)  [unwired: 2 in, 2 out]
    n19 = Dequeue Element(queue=w47) -> (element=w84:i16[], error out=w55:errorcluster)  [unwired: 2 in, 2 out]
    n20 = Dequeue Element(queue=w50) -> (element=w87:i16[], error out=w58:errorcluster)  [unwired: 2 in, 2 out]
    n21 = Dequeue Element(queue=w49) -> (element=w86:i16[], error out=w57:errorcluster)  [unwired: 2 in, 2 out]
    n22 = Dequeue Element(queue=w51) -> (element=w88:i16[], error out=w59:errorcluster)  [unwired: 2 in, 2 out]
    n23 = Tick Count (ms)() -> (millisecond timer value=w103:u32)
    n24 = Dequeue Element(queue=w52) -> (element=w89:i16[], error out=w60:errorcluster)  [unwired: 2 in, 2 out]
    n25 = Dequeue Element(queue=w107) -> (element=w108:i16[], error out=w61:errorcluster)  [unwired: 2 in, 2 out]
    n26 = Subtract(x=w103, y=w102) -> (x-y=w105:u32)
    n27 = case shown="No Error" w53 {
      tunnel: w94 -> [w139 w140]
      tunnel: [w138 w140] -> w93
      tunnel: w95 -> [w137 _]
      frame No Error {
        n28 = Build Array (concatenate)(w139, w137) -> (w138:i16[])
      }
      frame Error {
      }
    }
    n29 = case shown="No Error" w54 {
      tunnel: w72 -> [w111 w112]
      tunnel: [w110 w112] -> w62
      tunnel: w83 -> [w109 _]
      frame No Error {
        n30 = Build Array (concatenate)(w111, w109) -> (w110:i16[])
      }
      frame Error {
      }
    }
    n31 = case shown="No Error" w55 {
      tunnel: w73 -> [w115 w116]
      tunnel: [w114 w116] -> w63
      tunnel: w84 -> [w113 _]
      frame No Error {
        n32 = Build Array (concatenate)(w115, w113) -> (w114:i16[])
      }
      frame Error {
      }
    }
    n33 = Merge Errors(w61, w60, w59, w58, w57, w56, w55, w54, w53) -> (w90:errorcluster)
    n34 = case shown="No Error" w56 {
      tunnel: w74 -> [w119 w120]
      tunnel: [w118 w120] -> w64
      tunnel: w85 -> [w117 _]
      frame No Error {
        n35 = Build Array (concatenate)(w119, w117) -> (w118:i16[])
      }
      frame Error {
      }
    }
    n36 = case shown="No Error" w57 {
      tunnel: w75 -> [w123 w124]
      tunnel: [w122 w124] -> w65
      tunnel: w86 -> [w121 _]
      frame No Error {
        n37 = Build Array (concatenate)(w123, w121) -> (w122:i16[])
      }
      frame Error {
      }
    }
    n38 = case shown="No Error" w58 {
      tunnel: w76 -> [w127 w128]
      tunnel: [w126 w128] -> w66
      tunnel: w87 -> [w125 _]
      frame No Error {
        n39 = Build Array (concatenate)(w127, w125) -> (w126:i16[])
      }
      frame Error {
      }
    }
    n40 = case shown="No Error" w59 {
      tunnel: w79 -> [w131 w132]
      tunnel: [w130 w132] -> w77
      tunnel: w88 -> [w129 _]
      frame No Error {
        n41 = Build Array (concatenate)(w131, w129) -> (w130:i16[])
      }
      frame Error {
      }
    }
    n42 = case shown="No Error" w60 {
      tunnel: w82 -> [w135 w136]
      tunnel: [w134 w136] -> w80
      tunnel: w89 -> [w133 _]
      frame No Error {
        n43 = Build Array (concatenate)(w135, w133) -> (w134:i16[])
      }
      frame Error {
      }
    }
    n44 = case shown="No Error" w61 {
      tunnel: w106 -> [w214 w215]
      tunnel: [w213 w215] -> w99
      tunnel: w108 -> [w212 _]
      frame No Error {
        n45 = Build Array (concatenate)(w214, w212) -> (w213:i16[])
      }
      frame Error {
      }
    }
    n46 = Greater Or Equal?(x=w105, y=u32 1000) -> (x >= y?=w100:bool)
    n47 = Select(t=w103, s=w100, f=w102) -> (s? t:f=w101:u32)
    n48 = case shown="True" w100 {
      tunnel: w99 -> [w151 w161]
      tunnel: [w151 w158] -> w98
      tunnel: w97 -> [w150 w207]
      tunnel: [w150 w206] -> w96
      tunnel: w93 -> [w149 w152]
      tunnel: [w149 w158] -> w92
      tunnel: [w148 w205] -> w91
      tunnel: w90 -> [w148 w205]
      tunnel: [w147 w158] -> w81
      tunnel: w80 -> [w147 w160]
      tunnel: [w146 w158] -> w78
      tunnel: w77 -> [w146 w159]
      tunnel: [w145 w158] -> w71
      tunnel: [w144 w158] -> w70
      tunnel: [w143 w158] -> w69
      tunnel: [w142 w158] -> w68
      tunnel: [w141 w158] -> w67
      tunnel: w66 -> [w145 w157]
      tunnel: w65 -> [w144 w156]
      tunnel: w64 -> [w143 w155]
      tunnel: w63 -> [w142 w154]
      tunnel: w62 -> [w141 w153]
      frame False {
      }
      frame True {
        w174 = u16 0 items=["unsigned binary", "offset binary", "2's complement"] ("data format (offset binary)")
        w158 = i16[] [] ("History Data")
        # "Once a second, save accumulated data to disk. Use LV TDMS file\nfor best performance; standard binary write also works."
        n49 = local read "Max ADC value"() -> (w163:i16)
        n50 = local read "Channels"() -> (w162:T1)
        n51 = Unbundle By Name(w162) -> ("Channel H Settings.Range"=w192:u16)
        n52 = Unbundle By Name(w162) -> ("Channel G Settings.Range"=w193:u16)
        n53 = Unbundle By Name(w162) -> ("Channel A Settings.Range"=w203:u16)
        n54 = Unbundle By Name(w162) -> ("Channel D Settings.Range"=w196:u16)
        n55 = Unbundle By Name(w162) -> ("Channel E Settings.Range"=w195:u16)
        n56 = Unbundle By Name(w162) -> ("Channel F Settings.Range"=w194:u16)
        n57 = Unbundle By Name(w162) -> ("Channel B Settings.Range"=w202:u16)
        n58 = Unbundle By Name(w162) -> ("Channel C Settings.Range"=w197:u16)
        n59 = case shown="True" "Write ChA to file" {
          tunnel: w207 -> [w208 w211]
          tunnel: [w208 w210] -> w206
          tunnel: w161 -> [_ w209]
          frame False {
          }
          frame True {
            n60 = TDMS Write(0:w211, 9:w209) -> (4:w210:refnum<k34>)  [unwired: 4 in, 3 out]
          }
        }
        n61 = call "PicoScopeAdcToVolts.vi"("Max_adc"=w163, "Range Index"=w192, "Data"=w153) -> ("Data"=w189:dbl[])
        n62 = call "PicoScopeAdcToVolts.vi"("Max_adc"=w163, "Range Index"=w203, "Data"=w161) -> ("Data"=w201:dbl[])
        n63 = call "PicoScopeAdcToVolts.vi"("Max_adc"=w163, "Range Index"=w193, "Data"=w154) -> ("Data"=w183:dbl[])
        n64 = call "PicoScopeAdcToVolts.vi"("Max_adc"=w163, "Range Index"=w195, "Data"=w156) -> ("Data"=w186:dbl[])
        n65 = call "PicoScopeAdcToVolts.vi"("Max_adc"=w163, "Range Index"=w194, "Data"=w155) -> ("Data"=w182:dbl[])
        n66 = call "PicoScopeAdcToVolts.vi"("Max_adc"=w163, "Range Index"=w196, "Data"=w157) -> ("Data"=w187:dbl[])
        n67 = call "PicoScopeAdcToVolts.vi"("Max_adc"=w163, "Range Index"=w202, "Data"=w160) -> ("Data"=w200:dbl[])
        n68 = call "PicoScopeAdcToVolts.vi"("Max_adc"=w163, "Range Index"=w197, "Data"=w159) -> ("Data"=w188:dbl[])
        n69 = local read "DownSample Interval (sec)"() -> (w164:dbl)
        n70 = Bundle(0, "DownSample Interval (sec)"=w164, "Data"=w201) -> (w199:T9)  [unwired: 1 in]
        n71 = Bundle(0, "DownSample Interval (sec)"=w164, "Data"=w200) -> (w198:T9)  [unwired: 1 in]
        n72 = Bundle(0, "DownSample Interval (sec)"=w164, "Data"=w188) -> (w181:T9)  [unwired: 1 in]
        n73 = Bundle(0, "DownSample Interval (sec)"=w164, "Data"=w186) -> (w179:T9)  [unwired: 1 in]
        n74 = Bundle(0, "DownSample Interval (sec)"=w164, "Data"=w182) -> (w178:T9)  [unwired: 1 in]
        n75 = Bundle(0, "DownSample Interval (sec)"=w164, "Data"=w183) -> (w177:T9)  [unwired: 1 in]
        n76 = Bundle(0, "DownSample Interval (sec)"=w164, "Data"=w187) -> (w180:T9)  [unwired: 1 in]
        n77 = Bundle(0, "DownSample Interval (sec)"=w164, "Data"=w189) -> (w176:T9)  [unwired: 1 in]
        n78 = call-poly <vilib>:"Analog to Digital.vi"("data format (offset binary)"=w174, "full-scale range (pk-pk)"=256.0, "resolution (16 bit)"=8, "analog waveform"=w152) -> ("digital waveform"=w170:digitalwaveform)  [unwired: 4 in, 3 out]
        n79 = Build Array(w199, w198, w181, w180, w179, w178, w177, w176) -> (→"Analog Channels":T10)
        n80 = Bundle By Name("t0"=timestamp(0 s since 1904-01-01), "dt"=w164, "Y"=w170) -> (→"Port 0":digitalwaveform)  [unwired: 1 in]
      }
    }
  }
  n81 = Tick Count (ms)() -> (millisecond timer value=w36:u32)
  n82 = while {
    tunnel: w41 -> [w294]
    tunnel: [w262] -> w22
    tunnel: w37 -> [w216]
    tunnel: w26 -> [w292]
    tunnel: [w276] -> w25
    shift-right: [w261] -> w23
    shift-left: w40 -> [w293]
    tunnel: [w257] -> w24
    tunnel: w36 -> [w254]
    tunnel: w19 -> [w253]
    tunnel: w15 -> [w252]
    tunnel: [w251] -> w21
    tunnel: [w250] -> w20
    tunnel: T7 {"Max Buffer Pointers"=[], "Min Buffer Pointers"=[], "StreamingDataInfo"=[]} ("Data Pointers") -> [w249]
    tunnel: w14 -> [w248]
    tunnel: w13 -> [w247]
    tunnel: w12 -> [w246]
    tunnel: w11 -> [w245]
    tunnel: w10 -> [w244]
    tunnel: w9 -> [w243]
    tunnel: w8 -> [w242]
    tunnel: [w241] -> w7
    tunnel: [w240] -> w6
    tunnel: [w239] -> w5
    tunnel: [w238] -> w4
    tunnel: [w237] -> w3
    tunnel: [w236] -> w2
    tunnel: [w235] -> w1
    stop <- w270 stop-if-true
    w226 = 10.0 ("y")
    # "Calulate from SI units used"
    # "multiply by DownSample ratio"
    n83 = Unbundle By Name("Buffer and Transfer Settings") -> ("Samples"=w218:u64, "startIndex"=w219:u64)
    n84 = Subtract(x=w218, y=w219) -> (x-y=w217:u64)
    n85 = call "PicoScope6000aSettings.vi"("handle in"=w294, "Device Info"=w216, "Channels"="Channels", "Max ADC value"=w292, "error in (no error)"=w293, "Trigger Settings"="Trigger Settings", "Digital Channels"="Digital Channels") -> ("Enabled array"=w274:i16[], "handle out"=w288:i16, "error out"=w289:errorcluster)  [unwired: 6 in]
    n86 = feedback #1(w249) -> (w268:T7)
    n87 = call "PicoScope6000aSetupStreaming.vi"("handle in"=w288, "Streaming Acquisition Settings"="Streaming Acquisition Settings", "Buffer and Transfer Settings"="Buffer and Transfer Settings", "enabled array"=w274, "Device Info"=w216, "Data Pointers In"=w268, "Number of Buffers"="No of Buffers", "error in (no error)"=w289, "Auto Stop"="Auto Stop") -> ("handle out"=w281:i16, "Data Pointers"=w267:T7, "Actual sampleInterval"=w278:T11, "error out"=w280:errorcluster)  [unwired: 3 in]
    n88 = feedback-in #1(w267) -> ()
    n89 = Unbundle By Name(w278) -> ("sampleIntervalTimeUnits"=w284:u32, "sampleInterval"=w277:dbl)
    n90 = Tick Count (ms)() -> (millisecond timer value=w255:u32)
    n91 = Decrement(x="No of Buffers") -> (x-1=w256:i32)
    n92 = Multiply(x=3.0, y=w284) -> (x*y=w285:dbl)
    n93 = Power Of 10(x=w285) -> (10^x=w283:dbl)
    n94 = Divide(x=sgl 1000000000000000.0 ("y"), y=w283) -> (x/y=w282:dbl)
    n95 = Unbundle By Name("Buffer and Transfer Settings") -> ("Down-Sample Mode"=w263:u32, "Down Sample Ratio"=w264:u64)
    n96 = Divide(x=w277, y=w282) -> (x/y=w232:dbl)
    n97 = Multiply(x=w232, y=w217) -> (x*y=w220:dbl)
    n98 = Multiply(x=w220, y="Poll Holdoff %") -> (x*y=w224:dbl)
    n99 = Multiply(x=w220, y="Poll Delay %") -> (x*y=w225:dbl)
    n100 = Multiply(x=w224, y=w226) -> (x*y=w229:dbl)
    n101 = Multiply(x=w225, y=w226) -> (x*y=w230:dbl)
    n102 = To Unsigned Long Integer(number=w229) -> (unsigned 32bit integer=w227:u32)
    n103 = To Unsigned Long Integer(number=w230) -> (unsigned 32bit integer=w228:u32)
    n104 = Bundle(cluster=cluster{u32, u32} {0, 0}, w227, w228) -> (w231:cluster{u32, u32})
    n105 = case shown="80000000" w263 {
      tunnel: [w372 u64 1 ("Down Sample Ratio")] -> w290
      tunnel: w264 -> [w372 _]
      frame Default {
      }
      frame -2147483648 {
        # "No DownSampling"
      }
    }
    n106 = Multiply(x=w290, y=w232) -> (x*y=w234:dbl)
    "DownSample Interval (sec)" <- w234
    n107 = while {
      tunnel: w292 -> [_]
      tunnel: w234 -> [_]
      tunnel: "Buffer and Transfer Settings" -> [w351]
      tunnel: w281 -> [w358]
      tunnel: w274 -> [w352]
      tunnel: [w354] -> w259
      shift-right: [w353] -> w260
      shift-left: w280 -> [w359]
      shift-right: [w367] -> _
      shift-left: FALSE ("SetDataBuffer0") -> [w350]
      tunnel: [w352] -> w276
      tunnel: [w361] -> w271
      tunnel: w216 -> [w295]
      tunnel: w231 -> [w297]
      shift-right: [w329] -> _
      shift-left: 0 ("No of Buffers") -> [w347]
      shift-right: [w345] -> w257
      shift-left: w267 -> [w349]
      tunnel: w256 -> [w344]
      tunnel: w254 -> [w338]
      shift-right: [w337] -> _
      shift-left: w255 -> [w339]
      tunnel: w253 -> [w333]
      tunnel: w252 -> [w332]
      tunnel: [w331] -> w251
      tunnel: [w330] -> w250
      tunnel: w248 -> [w322]
      tunnel: w247 -> [w321]
      tunnel: w246 -> [w320]
      tunnel: w245 -> [w318]
      tunnel: w244 -> [w317]
      tunnel: w243 -> [w316]
      tunnel: w242 -> [w315]
      tunnel: [w314] -> w241
      tunnel: [w313] -> w240
      tunnel: [w312] -> w239
      tunnel: [w311] -> w238
      tunnel: [w310] -> w237
      tunnel: [w309] -> w236
      tunnel: [w308] -> w235
      stop <- w366 stop-if-true
      n108 = Unbundle By Name(w295) -> ("PICO_VARIANT_INFO"=w296:string)
      n109 = call "PicoScope6000aNextBuffer.vi"("handle in"=w358, "Buffer and Transfer Settings"=w351, "enabled array"=w352, "Device Info"=w295, "Data Pointers In"=w349, "Buffer Number"=w347, "error in (no error)"=w359, "LoopFlag"=w350) -> ("handle out"=w355:i16, "error out"=w357:errorcluster)  [unwired: 6 in]
      n110 = Equal?(x=w347, y=w344) -> (x = y?=w348:bool)
      n111 = case shown="False" w348 {
        tunnel: w347 -> [w370 _]
        tunnel: [w369 0] -> w329
        frame False {
          n112 = Increment(x=w370) -> (x+1=w369:i32)
        }
        frame True {
        }
      }
      n113 = call "PicoScope6000aGetStreamingLatestValues.vi"("handle in"=w355, "Polling Delays ms"=w297, "Buffer and Transfer Settings"=w351, "enabled array"=w352, "Device Info"=w295, "Data Pointers In"=w349, "Buffer number"=w347, "error in (no error)"=w357) -> ("handle out"=w354:i16, "Data Pointers Out"=w345:T7, "tPicoStreamingDataTriggerInfo"=w346:T12, "error out"=w356:errorcluster)  [unwired: 4 in]
      n114 = call "PicoReadPicoSingleBuffers.vi"("enabled array"=w352, "Buffer and Transfer Settings"=w351, "Variant"=w296, "Data Pointers"=w345, "Buffer Number"=w329, "error in (no error)"=w356) -> ("MaxBuffers (Max or non-aggregated)"=w299:T13, "error out"=w353:errorcluster)  [unwired: 7 in, 1 out]
      n115 = Unbundle By Name(w299) -> ("Channel A Buffer"=w298:i16[])
      n116 = Unbundle By Name(w299) -> ("Channel B Buffer"=w307:i16[])
      n117 = Unbundle By Name(w299) -> ("Channel C Buffer"=w306:i16[])
      n118 = Unbundle By Name(w299) -> ("Channel D Buffer"=w305:i16[])
      n119 = Unbundle By Name(w299) -> ("Channel G Buffer"=w302:i16[])
      n120 = Unbundle By Name(w299) -> ("Channel H Buffer"=w301:i16[])
      n121 = Unbundle By Name(w299) -> ("Channel E Buffer"=w304:i16[])
      n122 = Unbundle By Name(w299) -> ("Channel F Buffer"=w303:i16[])
      n123 = Unbundle By Name(w346) -> ("autoStop_"=w364:i16)
      n124 = Unbundle By Name(w299) -> ("Port 0 Buffer"=w300:i16[])
      n125 = Or(x=w350, y=TRUE) -> (x .or. y?=w367:bool)
      n126 = Not Equal To 0?(x=w364) -> (x != 0?=w363:bool)
      n127 = Tick Count (ms)() -> (millisecond timer value=w337:u32)
      n128 = Unbundle By Name(w353) -> ("status"=w360:bool)
      n129 = Subtract(x=w337, y=w338) -> (x-y=w341:u32)
      n130 = Subtract(x=w337, y=w339) -> (x-y=→"Chunk time":u32)
      n131 = Divide(x=w341, y=u32 1000) -> (x/y=→"Elapsed time":dbl)
      n132 = Compound Arithmetic op=OR(w363, "stop", w360) -> (w361:bool)
      n133 = Enqueue Element(queue=w333, element=w298) -> (queue out=w335:refnum<queue>)  [unwired: 2 in, 2 out]
      n134 = Enqueue Element(queue=w332, element=w307) -> (queue out=w334:refnum<queue>)  [unwired: 2 in, 2 out]
      n135 = Enqueue Element(queue=w322, element=w306) -> (queue out=w328:refnum<queue>)  [unwired: 2 in, 2 out]
      n136 = Enqueue Element(queue=w321, element=w305) -> (queue out=w327:refnum<queue>)  [unwired: 2 in, 2 out]
      n137 = Enqueue Element(queue=w320, element=w304) -> (queue out=w326:refnum<queue>)  [unwired: 2 in, 2 out]
      n138 = Enqueue Element(queue=w318, element=w303) -> (queue out=w323:refnum<queue>)  [unwired: 2 in, 2 out]
      n139 = Enqueue Element(queue=w317, element=w302) -> (queue out=w325:refnum<queue>)  [unwired: 2 in, 2 out]
      n140 = Enqueue Element(queue=w316, element=w301) -> (queue out=w324:refnum<queue>)  [unwired: 2 in, 2 out]
      n141 = Enqueue Element(queue=w315, element=w300) -> (queue out=w319:refnum<queue>)  [unwired: 2 in, 2 out]
      n142 = Get Queue Status(queue=w335) -> (queue out=w331:refnum<queue>, # elements in queue=→"queue depth" →"Queue depth":i32)  [unwired: 2 in, 6 out]
      n143 = Get Queue Status(queue=w334) -> (queue out=w330:refnum<queue>)  [unwired: 2 in, 7 out]
      n144 = Get Queue Status(queue=w328) -> (queue out=w314:refnum<queue>)  [unwired: 2 in, 7 out]
      n145 = Get Queue Status(queue=w327) -> (queue out=w313:refnum<queue>)  [unwired: 2 in, 7 out]
      n146 = Get Queue Status(queue=w326) -> (queue out=w312:refnum<queue>)  [unwired: 2 in, 7 out]
      n147 = Get Queue Status(queue=w323) -> (queue out=w311:refnum<queue>)  [unwired: 2 in, 7 out]
      n148 = Get Queue Status(queue=w325) -> (queue out=w310:refnum<queue>)  [unwired: 2 in, 7 out]
      n149 = Get Queue Status(queue=w324) -> (queue out=w309:refnum<queue>)  [unwired: 2 in, 7 out]
      n150 = Get Queue Status(queue=w319) -> (queue out=w308:refnum<queue>)  [unwired: 2 in, 7 out]
      n151 = Compound Arithmetic op=OR(w361, "Apply Settings", w360) -> (w366:bool)
    }
    n152 = call "PicoScope6000aStop.vi"("error in (no error)"=w260, "handle in"=w259) -> ("error out"=w261:errorcluster, "handle out"=w262:i16)  [unwired: 8 in]
    n153 = Unbundle By Name(w261) -> ("status"=w272:bool)
    n154 = Or(x=w271, y=w272) -> (x .or. y?=w270:bool)
  }
  n155 = flat-sequence {
    tunnel: w25 -> [w377]
    tunnel: w24 -> [w376]
    tunnel: w23 -> [w375]
    tunnel: w22 -> [w374]
    tunnel: w21 -> [w387]
    tunnel: w20 -> [w386]
    tunnel: w7 -> [w385]
    tunnel: w6 -> [w384]
    tunnel: w5 -> [w383]
    tunnel: w4 -> [w382]
    tunnel: w3 -> [w381]
    tunnel: w2 -> [w380]
    tunnel: w1 -> [w379]
    frame #0 {
      n156 = call "PicoScope6000aClose.vi"("error in (no error)"=w375, "handle in"=w374) -> ("error out"=w378:errorcluster)  [unwired: 8 in, 1 out]
      n157 = call "PicoReleaseMultiBuffers.vi"("error in (no error)"=w378, "Enabled array"=w377, "Data Pointers"=w376) -> ()  [unwired: 8 in, 1 out]
    }
    frame #1 {
      n158 = Release Queue(queue=w387) -> ()  [unwired: 2 in, 3 out]
      n159 = Release Queue(queue=w386) -> ()  [unwired: 2 in, 3 out]
      n160 = Release Queue(queue=w385) -> ()  [unwired: 2 in, 3 out]
      n161 = Release Queue(queue=w384) -> ()  [unwired: 2 in, 3 out]
      n162 = Release Queue(queue=w383) -> ()  [unwired: 2 in, 3 out]
      n163 = Release Queue(queue=w382) -> ()  [unwired: 2 in, 3 out]
      n164 = Release Queue(queue=w381) -> ()  [unwired: 2 in, 3 out]
      n165 = Release Queue(queue=w380) -> ()  [unwired: 2 in, 3 out]
      n166 = Release Queue(queue=w379) -> ()  [unwired: 2 in, 3 out]
    }
  }
  n167 = TDMS Close(11:w32) -> ()  [unwired: 1 in, 2 out]
